vi "CPP_SpectraFit.vi"() -> (5 "Plug in titles":string[](array[string]), 7 "Plug in values":string[](array[string]))   [LabVIEW 2016]
uses:
  <vilib>/Analysis/2dsp.llb/Integral Method.ctl
  Controls/Instrument_Array.ctl
  Controls/Post_Process.ctl
  Controls/Graph_Type.ctl
  <vilib>/Analysis/8numeric.llb/1D Numeric Integration.vi
  Globals/Meas_global.vi
  <vilib>/Analysis/NI_AALPro.lvlib
  <vilib>/Analysis/NI_AALBase.lvlib
panel:
  out "mean":dbl format="%0.2f"
  out "variance":dbl format="%.4f"
  out "Integral":dbl format="%0.4f"
  in  "integration method":T1 items=["Trapezoidal Rule", "Simpson's Rule", "Simpson's 3/8 Rule", "Bode Rule"]
  in  "Divider":i32(slide)=10 scale=1.0..100000.0 scale format="%#_6e"
  out "dF/ Hz":dbl
  in  "Show Smooth":bool=TRUE
  in  "Save Spectra?":bool
  in  "Desired number of samples per block":i32=32768
  out "Spectra":cluster{"Frequencies":dbl[], dbl[]}[](graph)
  in  "Averaging samples":i32=1 min=1 max=1000
  in  "Spectra Index (from ALL channels)":i32
  out "Waveform Graph":dbl[][](graph)
  in  "Channels to Plot":i32[](array[ring])=[0] items=["Pitot (URef)", "Mano (5HP1)", "Mano (5HP2)", "Mano (5HP3)", "Mano (5HP4)", "Mano (5HP5)", "HW (Uhf)", "Save Nothing"]
  # "Run this VI to update the channel names"
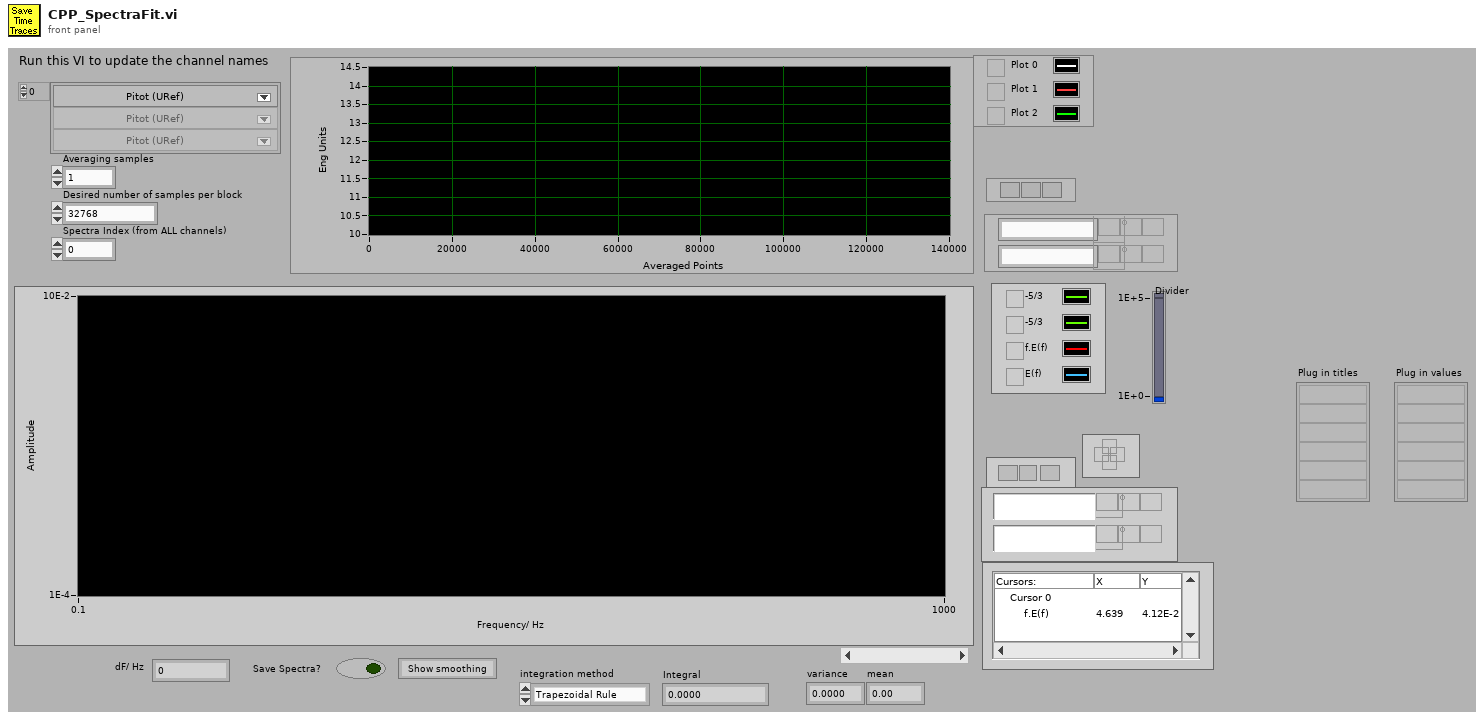
[diagram p1: front panel]
types:
  T1 = typedef "NI_AALPro.lvlib/Integral Method.ctl" = i32
  T2 = typedef "Analysis_info_cluster.ctl" = cluster{"Colour":u32, "Inst type":T3, "Inst name":string, "Symbol":string, "Code name":string, "Extra Info":string, "Inst Array":T4, "Extra Titles":string[], "Extra Values":string[], "U":dbl, "u^2":dbl, "u^3":dbl, "u^4":dbl, "Skew_u":dbl, "Kurt_u":dbl, "Sd Error in Mean":dbl, "% u'/U":dbl, "X":dbl, "Y":dbl, "Z":dbl, "Timescale integral to 25%":dbl, "Sd Error in Variance":dbl, "Calib File":path, "Calib Constants":dbl[], "Output Position":bool, "Full Stats":bool, "Av Sampling Rate":dbl, "Av No of Samples":dbl, "Total Meas Time (s)":dbl, "ADAM Ch Name":string, "Max value":dbl, "Min value":dbl}
  T3 = typedef "Inst_type.ctl" = enum16{"Propeller anemometer", "Raw voltage", "Pressure Transducer", "Pitot-static tube", "Preston tube", "Hot wire", "Cross wire 1", "Cross wire 2", "Generic Linear", "Generic Polynomial", "Generic BackPoly", "Fast FID", "Thermocouple", "Cold wire", "Pulsed Wire", "LDA Vel", "LDA Tran time", "LDA Arr time", "Microphone"}
  T4 = typedef "Instrument_Array.ctl" = enum16{"PWA", "LDA", "Analogue"}
  T5 = typedef "Post_Process.ctl" = enum16{"Take New Data", "Post Process Raw Data File"}
  T6 = typedef "Graph_Type.ctl" = enum16{"Show no graph", "Voltage trace", "Velocity trace", "Vel histogram", "Spectrum", "f.E(f) v Log f", "Auto-Corr"}
  T7 = cluster{"Plot 1":u16, "Plot 2":u16, "Save graph":u16, "Plot Type":T6}
  T8 = typedef "Time_Trace_Cluster.ctl" = cluster{"Weighting":dbl[], "Time (s)":dbl[], "Voltage":dbl[], "Eng Values":dbl[]}
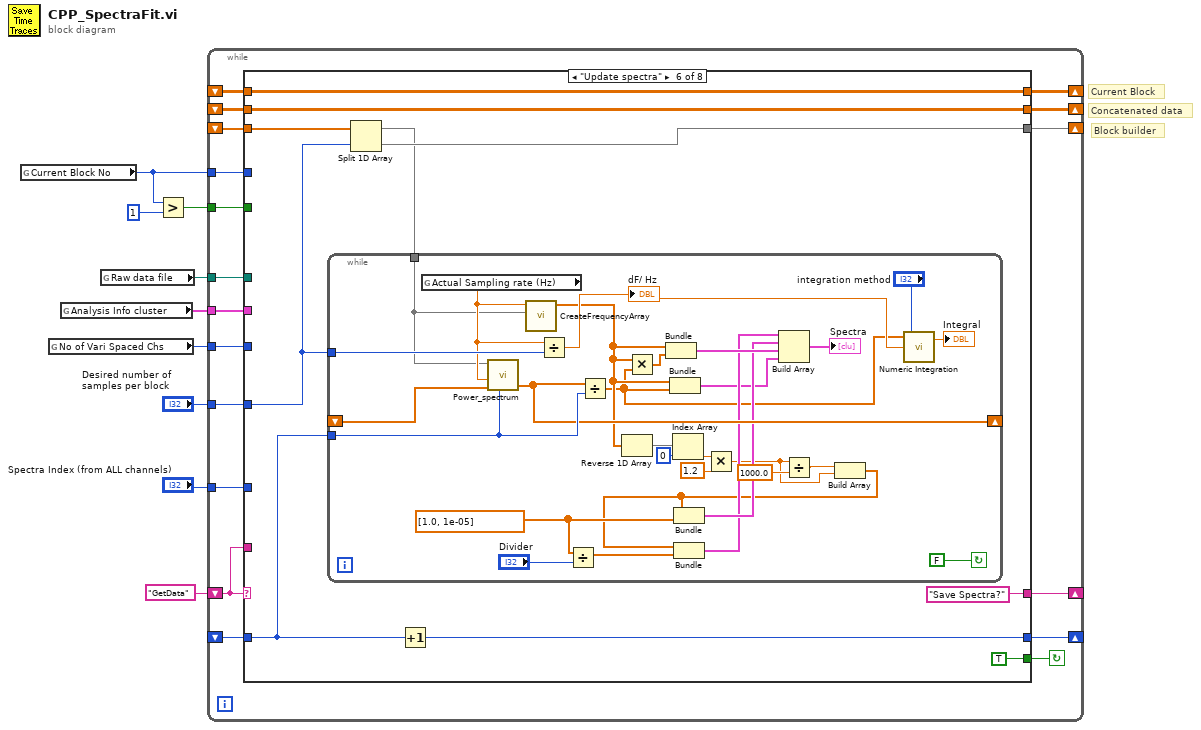
[diagram p0: block diagram]
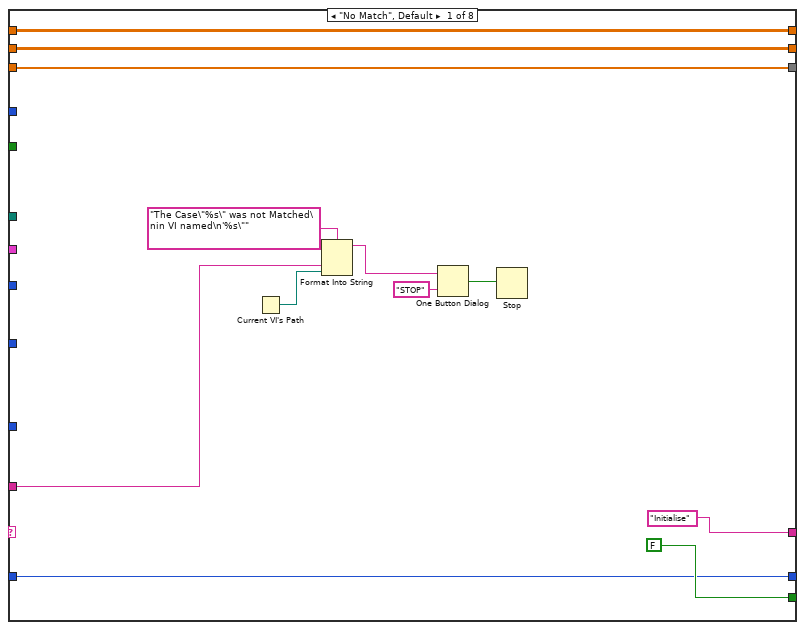
[diagram p2: hidden frame]
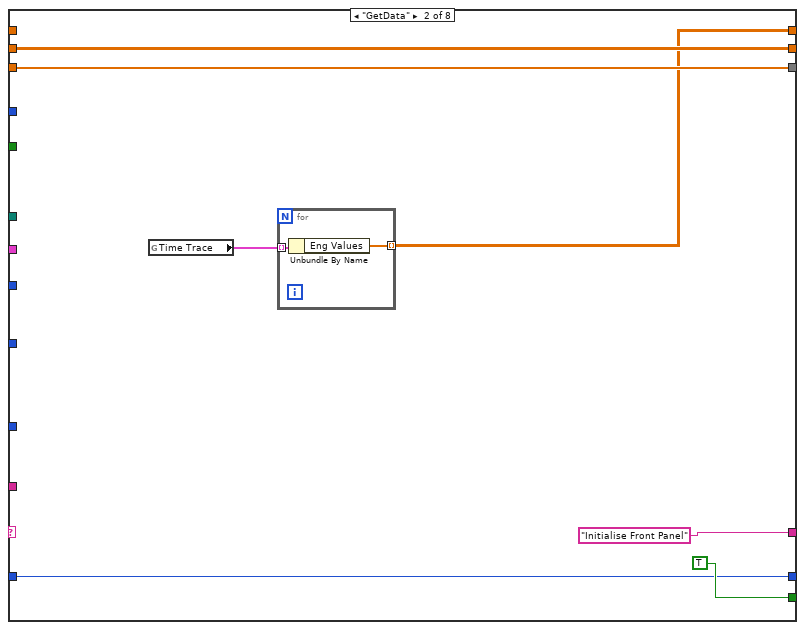
[diagram p3: hidden frame]
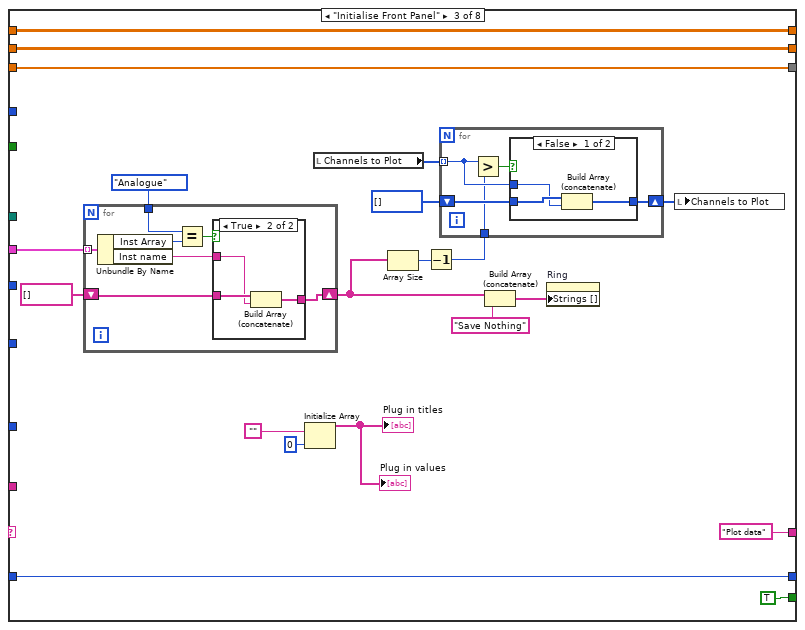
[diagram p4: hidden frame]
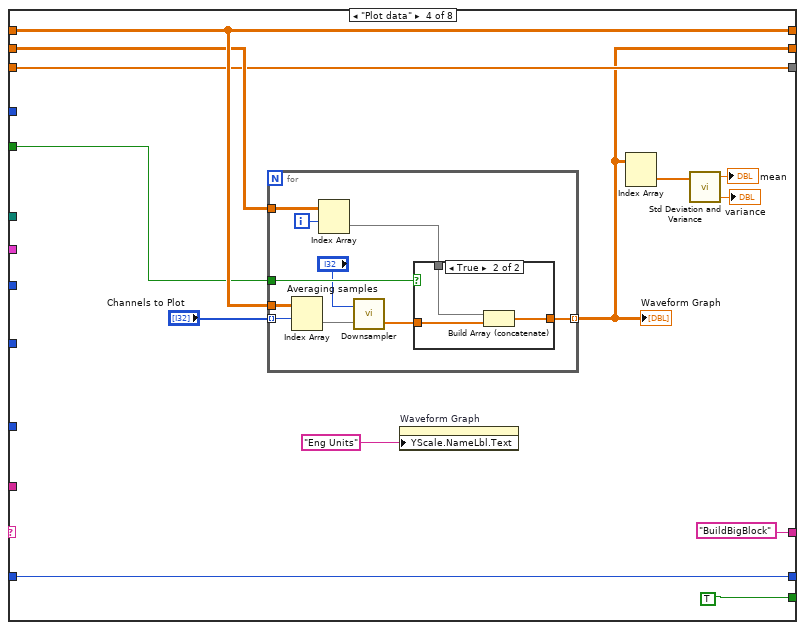
[diagram p7: hidden frame]
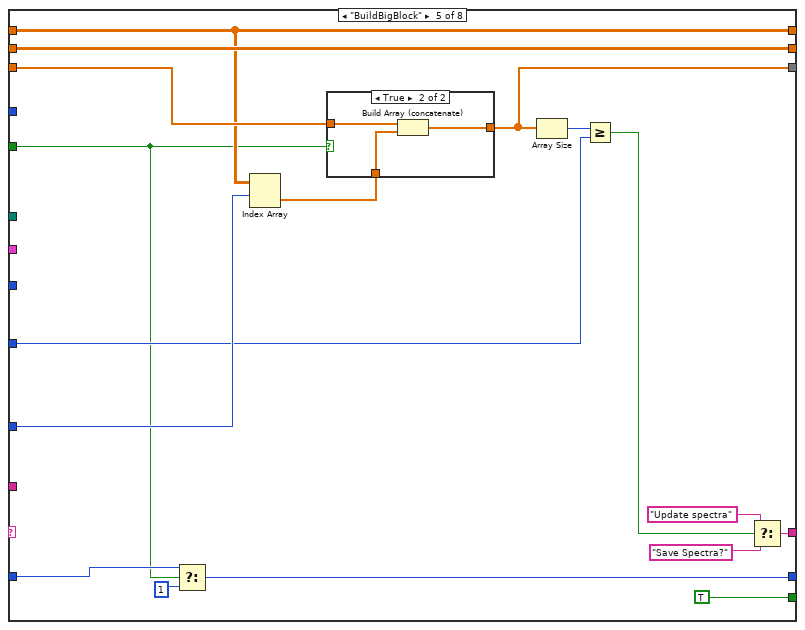
[diagram p9: hidden frame]
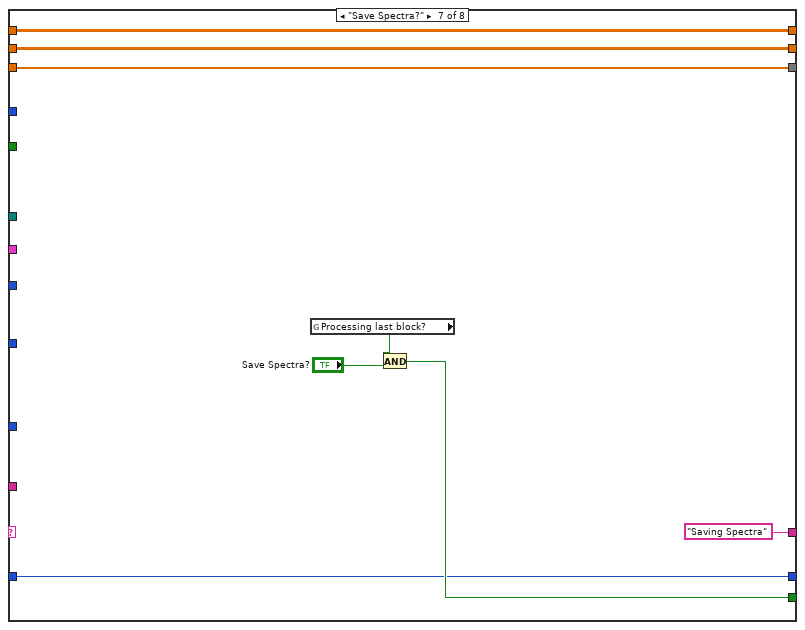
[diagram p11: hidden frame]
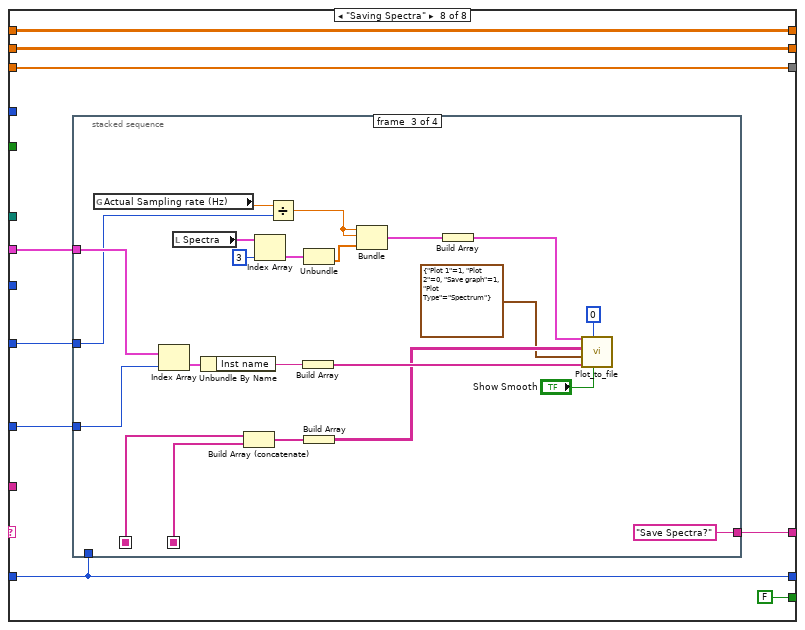
[diagram p12: hidden frame]
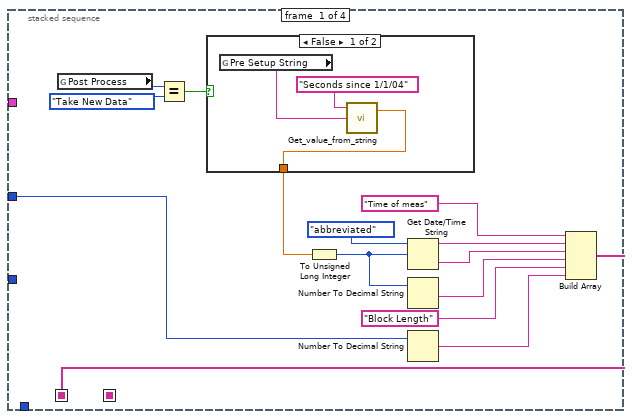
[diagram p13: hidden frame]
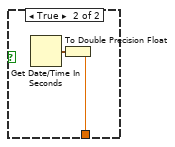
[diagram p14: hidden frame]
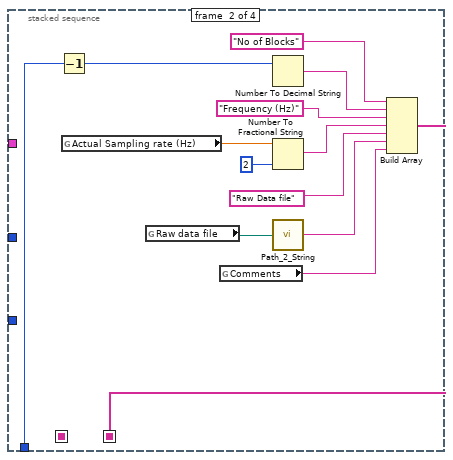
[diagram p15: hidden frame]
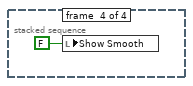
[diagram p16: hidden frame]
diagram:
  # "Block builder"
  # "Concatenated data"
  # "Current Block"
  n1 = global read "Meas_global.vi" "Current Block No"() -> (w6:i32)
  n2 = global read "Meas_global.vi" "No of Vari Spaced Chs"() -> (w4:i32)
  n3 = global read "Meas_global.vi" "Analysis Info cluster"() -> (w5:T2[])
  n4 = global read "Meas_global.vi" "Raw data file"() -> (w8:path)
  n5 = Greater?(x=w6, y=1) -> (0:w3:bool)
  n6 = while {
    shift-left: "GetData" -> [w25]
    shift-right: [w26] -> _
    tunnel: w8 -> [w24]
    tunnel: w3 -> [w23]
    tunnel: w6 -> [w22]
    tunnel: w5 -> [w21]
    tunnel: w4 -> [w20]
    shift-right: [w19] -> _
    shift-left: _ -> [w18]
    shift-right: [w16] -> _
    shift-left: _ -> [w17]
    shift-right: [w14] -> _
    shift-left: _ -> [w15]
    tunnel: "Desired number of samples per block" -> [w13]
    tunnel: "Spectra Index (from ALL channels)" -> [w12]
    shift-right: [w11] -> _
    shift-left: _ -> [w10]
    stop <- w27 continue-if-true
    n7 = case shown="\"Update spectra\"" w25 {
      tunnel: [FALSE TRUE TRUE TRUE ("Calculate Spectra and Histogram?") TRUE ("Calculate Spectra and Histogram?") TRUE ("Calculate Spectra and Histogram?") w177 FALSE ("Calculate Spectra and Histogram?")] -> w27
      tunnel: ["Initialise" "Initialise Front Panel" "Plot data" "BuildBigBlock" ("t") w117 "Save Spectra?" "Saving Spectra" w190] -> w26
      tunnel: w25 -> [w34 _ _ _ _ _ _ _]
      tunnel: w24 -> [_ _ _ _ _ _ _ _]
      tunnel: w23 -> [_ _ _ w99 w120 _ _ _]
      tunnel: w22 -> [_ _ _ _ _ _ _ _]
      tunnel: w21 -> [_ _ w52 _ _ _ _ w188]
      tunnel: w20 -> [_ _ _ _ _ _ _ _]
      tunnel: [w31 w40 w58 w101 w130 w145 w182 w191] -> w19
      tunnel: w18 -> [w31 _ w58 w101 w130 w145 w182 w191]
      tunnel: w17 -> [w30 w44 w57 w100 w131 w146 w183 w192]
      tunnel: [w30 w44 w57 w92 w131 w146 w183 w192] -> w16
      tunnel: w15 -> [w29 w43 w54 w96 w132 w144 w180 w189]
      tunnel: [w29 w43 w54 w96 w128 w143 w180 w189] -> w14
      tunnel: w13 -> [_ _ _ _ w124 w139 _ w185]
      tunnel: w12 -> [_ _ _ _ w126 _ _ w187]
      tunnel: [w28 w42 w53 w95 w121 w137 w176 w184] -> w11
      tunnel: w10 -> [w28 w42 w53 w95 w122 w138 w176 w184]
      frame "No Match", Default {
        n8 = Current VI's Path() -> (path=w33:path)
        n9 = Format Into String(format string="The Case\"%s\" was not Matched\nin VI named\n'%s\"" ("Format String"), w34, w33) -> (resulting string=w37:string)  [unwired: 2 in, 1 out]
        n10 = One Button Dialog(message=w37, button name ("OK")="STOP") -> (true=w35:bool)
        n11 = Stop(stop? (T)=w35) -> ()
      }
      frame "GetData" {
        n12 = global read "Meas_global.vi" "Time Trace"() -> (w41:T8[])
        n13 = for {
          tunnel: w41 -> [w48] mode=indexing
          tunnel: [w47] -> w40 mode=indexing
          n14 = Unbundle By Name(w48) -> ("Eng Values"=w47:dbl[])
        }
      }
      frame "Initialise Front Panel" {
        n15 = for {
          tunnel: Instrument_Array."Analogue" ("Inst Array") -> [w74]
          tunnel: w52 -> [w73] mode=indexing
          shift-right: [w70] -> w51
          shift-left: string[] [] -> [w71]
          n16 = Unbundle By Name(w73) -> ("Inst Array"=w75:T4, "Inst name"=w69:string)
          n17 = Equal?(x=w74, y=w75) -> (x = y?=w72:bool)
          n18 = case shown="True" w72 {
            tunnel: w71 -> [w76 w79]
            tunnel: [w76 w78] -> w70
            tunnel: w69 -> [_ w77]
            frame False {
            }
            frame True {
              n19 = Build Array (concatenate)(w79, w77) -> (w78:string[])
            }
          }
        }
        n20 = Initialize Array("", 0) -> (→"Plug in values" →"Plug in titles":string[])
        n21 = local read "Channels to Plot"() -> (w65:i32[])
        n22 = Array Size(array=w51) -> (size(s)=w60:i32)
        n23 = Decrement(x=w60) -> (x-1=w59:i32)
        n24 = for {
          tunnel: w65 -> [w81] mode=indexing
          shift-right: [w82] -> w63
          shift-left: i32[] [] -> [w83]
          tunnel: w59 -> [w80]
          n25 = Greater?(x=w81, y=w80) -> (0:w84:bool)
          n26 = case shown="False" w84 {
            tunnel: w83 -> [w87 w88]
            tunnel: [w86 w88] -> w82
            tunnel: w81 -> [w85 _]
            frame False {
              n27 = Build Array (concatenate)(w87, w85) -> (w86:i32[])
            }
            frame True {
            }
          }
        }
        n28 = Build Array (concatenate)(w51, "Save Nothing") -> (w61:string[])
        n29 = property on="Ring" class="Ring (strict)"("Strings []"=w61) -> ()  [unwired: 2 in, 2 out]
        n30 = local write "Channels to Plot"(w63) -> ()
      }
      frame "Plot data" {
        n31 = for {
          tunnel: w101 -> [w111]
          tunnel: "Channels to Plot" -> [w110] mode=indexing
          tunnel: w100 -> [w107]
          tunnel: [w108] -> w92 mode=indexing
          tunnel: w99 -> [w109]
          i -> [w106]
          n32 = Index Array(array=w111, index (row)=w110) -> (element=w104:dbl[])  [unwired: 1 in]
          n33 = Index Array(array=w107, index (row)=w106) -> (element=w105:dbl[])  [unwired: 1 in]
          n34 = call "Downsampler.vi"("Input Array"=w104, "Averaging samples"="Averaging samples") -> ("Downsampled Array"=w103:dbl[])  [unwired: 1 out]
          n35 = case shown="True" w109 {
            tunnel: w105 -> [_ w115]
            tunnel: w103 -> [w112 w114]
            tunnel: [w112 w113] -> w108
            frame False {
            }
            frame True {
              n36 = Build Array (concatenate)(w115, w114) -> (w113:dbl[])
            }
          }
        }
        "Waveform Graph" <- w92
        n37 = property on="Waveform Graph" class="WFGraph (strict)"("YScale.NameLbl.Text"="Eng Units") -> ()  [unwired: 2 in, 2 out]
        n38 = Index Array(array=w92) -> (element=w91:dbl[])  [unwired: 2 in]
        n39 = call <vilib>:"Std Deviation and Variance.vi"("X"=w91) -> ("mean"=→"mean":dbl, "variance"=→"variance":dbl)  [unwired: 1 in, 1 out]
      }
      frame "BuildBigBlock" {
        n40 = Select(t=w122, s=w120, f=1) -> (s? t:f=w121:i32)
        n41 = Index Array(array=w130, index (row)=w126) -> (element=w129:dbl[])  [unwired: 1 in]
        n42 = case shown="True" w120 {
          tunnel: w132 -> [_ w136]
          tunnel: [w133 w135] -> w128
          tunnel: w129 -> [w133 w134]
          frame False {
          }
          frame True {
            n43 = Build Array (concatenate)(w136, w134) -> (w135:dbl[])
          }
        }
        n44 = Array Size(array=w128) -> (size(s)=w127:i32)
        n45 = Greater Or Equal?(x=w127, y=w124) -> (x >= y?=w116:bool)
        n46 = Select(t="Update spectra", s=w116, f="Save Spectra?") -> (s? t:f=w117:string)
      }
      frame "Update spectra" {
        n47 = Split 1D Array(array=w144, index=w139) -> (first subarray=w140:dbl[], second subarray=w143:dbl[])
        n48 = while {
          shift-left: _ -> [w171]
          shift-right: [w172] -> _
          tunnel: w140 -> [w169]
          tunnel: w138 -> [w174]
          tunnel: w139 -> [w173]
          stop <- FALSE continue-if-true
          w164 = dbl[] [1.0, 1e-05]
          n49 = global read "Meas_global.vi" "Actual Sampling rate (Hz)"() -> (w170:dbl)
          n50 = call "Power_spectrum.vi"("U"=w169, "Sampling frequency"=w170, "Spectrum input array"=w171, "Block No"=w174) -> ("Spectrum Accumulator array"=w172:dbl[])  [unwired: 1 in, 2 out]
          n51 = call "CreateFrequencyArray.vi"("Signal"=w169, "Actual Sampling rate (Hz)"=w170) -> ("Frequencies"=w150:dbl[])  [unwired: 9 in]
          n52 = Divide(x=w170, y=w173) -> (x/y=w151:dbl)
          "dF/ Hz" <- w151
          n53 = Divide(x=w164, y="Divider") -> (x/y=w165:dbl[])
          n54 = Divide(x=w172, y=w174) -> (x/y=w147:dbl[])
          n55 = Reverse 1D Array(array=w150) -> (reversed array=w159:dbl[])
          n56 = Multiply(x=w150, y=w147) -> (x*y=w161:dbl[])
          n57 = Bundle("Frequencies"=w150, w161) -> (w167:cluster{"Frequencies":dbl[], dbl[]})  [unwired: 1 in]
          n58 = Bundle("Frequencies"=w150, w147) -> (w160:cluster{"Frequencies":dbl[], dbl[]})  [unwired: 1 in]
          n59 = Index Array(array=w159, index=0) -> (element=w157:dbl)
          n60 = Multiply(x=w157, y=1.2) -> (x*y=w153:dbl)
          n61 = Divide(x=w153, y=1000.0) -> (x/y=w154:dbl)
          n62 = Build Array(w154, w153) -> (w152:dbl[])
          n63 = Bundle(w152, w164) -> (w166:cluster{dbl[], dbl[]})  [unwired: 1 in]
          n64 = Bundle(w152, w165) -> (w162:cluster{dbl[], dbl[]})  [unwired: 1 in]
          n65 = Build Array(w162, w166, w167, w160) -> (→"Spectra":cluster{"Frequencies":dbl[], dbl[]}[])
          n66 = call-poly <vilib>:"Numeric Integration.vi"("integration method"="integration method", "dt"=w151, "Input Array"=w147) -> ("result"=→"Integral":dbl)  [unwired: 1 out]
        }
        n67 = Increment(x=w138) -> (x+1=w137:i32)
      }
      frame "Save Spectra?" {
        n68 = global read "Meas_global.vi" "Processing last block?"() -> (w178:bool)
        n69 = And(x=w178, y="Save Spectra?") -> (x .and. y?=w177:bool)
      }
      frame "Saving Spectra" {
        n70 = stacked-sequence {
          seq-local: [w196 _ _ _] -> [_ _ w238 _]
          seq-local: [_ w216 _ _] -> [_ _ w237 _]
          tunnel: [_ _ "Save Spectra?" _] -> w190
          tunnel: w188 -> [_ _ w244 _]
          tunnel: w187 -> [_ _ w243 _]
          tunnel: w185 -> [w194 _ w229 _]
          tunnel: w184 -> [_ w214 _ _]
          frame #0 {
            n71 = global read "Meas_global.vi" "Post Process"() -> (w198:T5)
            n72 = Equal?(x=w198, y=Post_Process."Take New Data" ("Post Process")) -> (x = y?=w199:bool)
            n73 = case shown="False" w199 {
              tunnel: [w207 w211] -> w200
              frame False {
                n74 = global read "Meas_global.vi" "Pre Setup String"() -> (w208:string)
                n75 = call "Get_value_from_string.vi"("Input string"=w208, "Variable name"="Seconds since 1/1/04") -> ("Value"=w207:dbl)  [unwired: 1 in, 1 out]
              }
              frame True {
                n76 = Get Date/Time In Seconds() -> (seconds since 1Jan1904=w210:timestamp)
                n77 = To Double Precision Float(number=w210) -> (double precision float=w211:dbl)
              }
            }
            n78 = To Unsigned Long Integer(number=w200) -> (unsigned 32bit integer=w204:u32)
            n79 = Get Date/Time String(date format (0)=enum16{"short", "long", "abbreviated"}."abbreviated", seconds (now)=w204) -> (date string=w202:string, time string=w203:string)  [unwired: 1 out]
            n80 = Number To Decimal String(number=w204) -> (decimal integer string=w205:string)  [unwired: 1 out]
            n81 = Number To Decimal String(number=w194) -> (decimal integer string=w193:string)  [unwired: 1 out]
            n82 = Build Array("Time of meas", w202, w203, w205, "Block Length" ("element"), w193) -> (w196:string[])
          }
          frame #1 {
            n83 = Decrement(x=w214) -> (x-1=w213:i32)
            n84 = global read "Meas_global.vi" "Actual Sampling rate (Hz)"() -> (w217:dbl)
            n85 = global read "Meas_global.vi" "Raw data file"() -> (w223:path)
            n86 = global read "Meas_global.vi" "Comments"() -> (w222:string)
            n87 = Number To Decimal String(number=w213) -> (decimal integer string=w212:string)  [unwired: 1 out]
            n88 = Number To Fractional String(number=w217, precision (6)=i16 2) -> (F-format string=w220:string)  [unwired: 2 out]
            n89 = call "Path_2_String.vi"("Real Path"=w223) -> ("Path String"=w224:string)
            n90 = Build Array("No of Blocks", w212, "Frequency (Hz)", w220, "Raw Data file", w224, w222) -> (w216:string[])
          }
          frame #2 {
            n91 = global read "Meas_global.vi" "Actual Sampling rate (Hz)"() -> (w230:dbl)
            n92 = Index Array(array=w244, index=w243) -> (element=w242:T2)
            n93 = local read "Spectra"() -> (w233:cluster{"Frequencies":dbl[], dbl[]}[])
            n94 = Unbundle By Name(w242) -> ("Inst name"=w241:string)
            n95 = Build Array (concatenate)(w238, w237) -> (w236:string[])
            n96 = Index Array(array=w233, index=3) -> (element=w231:cluster{"Frequencies":dbl[], dbl[]})
            n97 = Divide(x=w230, y=w229) -> (x/y=w227:dbl)
            n98 = Build Array(w241) -> (w240:string[])
            n99 = Unbundle(w231) -> (w228:dbl[])  [unwired: 1 out]
            n100 = Build Array(w236) -> (w235:string[][])
            n101 = Bundle(w227, w227, w228) -> (w226:cluster{dbl, dbl, dbl[]})  [unwired: 1 in]
            n102 = Build Array(w226) -> (w225:cluster{dbl, dbl, dbl[]}[])
            n103 = call "Plot_to_file.vi"("Show Smooth"="Show Smooth", "Start trace No"=0, "Trace names"=w240, "Graph"=T7 {"Plot 1"=1, "Plot 2"=0, "Save graph"=1, "Plot Type"=enum."Spectrum"}, "Plot file label"=w235, "Plot data"=w225) -> ()  [unwired: 6 out]
          }
          frame #3 {
            n104 = local write "Show Smooth"(FALSE ("Show Smooth")) -> ()
          }
        }
      }
    }
  }
